vi "Kaelus PIM MeasParams TCP Cmds.vi"(1 "Option D?":bool, 4 "Legacy (f)?":bool, 6 "Force?":bool, 8 "error in":errorcluster, 9 "Measurement Parameters":T1={"IM Order"=0, "Averaging"=1, "Direction"=0, "Enable ALC?"=FALSE, "Enable SingleIM?"=FALSE, "Display Units"=enum."dBm", "VA Hold?"=FALSE, "DUT PORT"=enum."Port 1"} {"Direction" items=["Reverse", "Forward", "Auxiliary"]; "IM Order" items=["3rd", "5th", "7th", "9th", "11th", "13th", "15th", "17th", "19th", "21st", "23rd", "25th", "27th", "29th", "31st", "33rd"]; "Averaging" items=["None", "Minimum", "Normal", "High", "Maximum"]}) -> (0 "error out":errorcluster)   [LabVIEW 2011]
uses:
  PIM Cmd Params.ctl
  BPIMCore/HW IO/IMOrder.ctl
  BPIMCore/HW IO/HW Averaging.ctl
  BPIMCore/HW IO/MeasMode.ctl
  BPIMCore/Display/display_unit_format.ctl
  BPIMCore/HW IO/DUTport.ctl
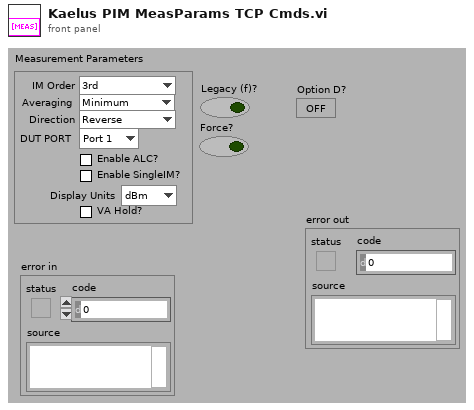
[diagram p1: front panel]
types:
  T1 = typedef "PIM Cmd Params.ctl" = cluster{"IM Order":T2, "Averaging":T3, "Direction":T4, "Enable ALC?":bool, "Enable SingleIM?":bool, "Display Units":T5, "VA Hold?":bool, "DUT PORT":T6}
  T2 = typedef "IMOrder.ctl" = u8
  T3 = typedef "HW Averaging.ctl" = u16
  T4 = typedef "MeasMode.ctl" = u16
  T5 = typedef "display_unit_format.ctl" = enum16{"dBm", "dBc"}
  T6 = typedef "DUTport.ctl" = enum16{"Port 1", "Port 2"}
  T7 = typedef "PIM.API.Command.Unique.ctl" = cluster{"#attributes":cluster{"Action":string}, "Double":dbl[], "Integer":i32[], "Boolean":bool[], "String":string[]}
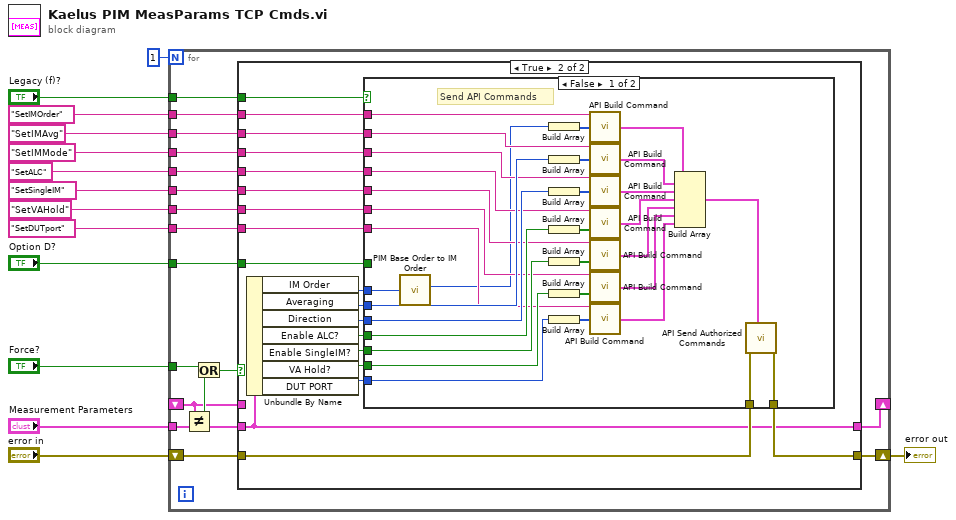
[diagram p0: block diagram]
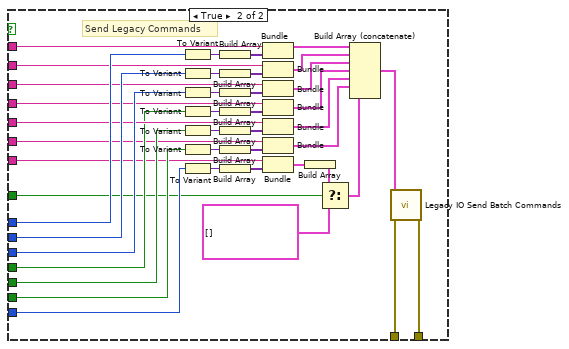
[diagram p3: hidden frame]
diagram:
  n1 = for {
    N: 1 -> [_]
    tunnel: "SetIMOrder" -> [w31]
    tunnel: "SetIMAvg" -> [w30]
    tunnel: "SetIMMode" -> [w29]
    tunnel: "SetALC" -> [w28]
    tunnel: "SetSingleIM" -> [w27]
    tunnel: "SetVAHold" -> [w26]
    tunnel: "SetDUTport" -> [w25]
    tunnel: "Option D?" -> [w24]
    shift-right: [w22] -> w5
    shift-left: "error in" -> [w23]
    shift-right: [w17] -> _
    shift-left: _ -> [w16]
    tunnel: "Measurement Parameters" -> [w19]
    tunnel: "Force?" -> [w20]
    tunnel: "Legacy (f)?" -> [w15]
    n2 = Not Equal?(x=w16, y=w19) -> (x != y?=w21:bool)
    n3 = Or(x=w20, y=w21) -> (x .or. y?=w18:bool)
    n4 = case shown="True" w18 {
      tunnel: w31 -> [_ w51]
      tunnel: w30 -> [_ w50]
      tunnel: w29 -> [_ w48]
      tunnel: w28 -> [_ w46]
      tunnel: w27 -> [_ w45]
      tunnel: w26 -> [_ w41]
      tunnel: w25 -> [_ w39]
      tunnel: w24 -> [_ w38]
      tunnel: w23 -> [w32 w37]
      tunnel: [w32 w36] -> w22
      tunnel: w19 -> [_ w35]
      tunnel: [w33 w35] -> w17
      tunnel: w16 -> [w33 _]
      tunnel: w15 -> [_ w34]
      frame False {
        # "No Changes have been made, proceed without sending commands."
      }
      frame True {
        n5 = Unbundle By Name(w35) -> ("IM Order"=w52:T2, "Averaging"=w49:T3, "Direction"=w47:T4, "Enable ALC?"=w44:bool, "Enable SingleIM?"=w43:bool, "VA Hold?"=w42:bool, "DUT PORT"=w40:T6)
        n6 = case shown="False" w34 {
          tunnel: w52 -> [w54 w126]
          tunnel: w51 -> [w84 w124]
          tunnel: w50 -> [w82 w121]
          tunnel: w49 -> [w81 w119]
          tunnel: w48 -> [w69 w117]
          tunnel: w47 -> [w79 w115]
          tunnel: w46 -> [w68 w113]
          tunnel: w45 -> [w67 w110]
          tunnel: w44 -> [w78 w108]
          tunnel: w43 -> [w77 w107]
          tunnel: w42 -> [w76 w106]
          tunnel: w41 -> [w66 w103]
          tunnel: w40 -> [w75 w102]
          tunnel: w39 -> [w65 w101]
          tunnel: w38 -> [_ w91]
          tunnel: w37 -> [w64 w86]
          tunnel: [w63 w85] -> w36
          frame False {
            # "Send API Commands"
            n7 = call "PIM Base Order to IM Order.vi"("Base Order (0)"=w54) -> ("IM Order"=w53:u8)  [unwired: 4 in, 1 out]
            n8 = Build Array(w53) -> (w83:u8[])
            n9 = Build Array(w81) -> (w80:T3[])
            n10 = Build Array(w79) -> (w70:T4[])
            n11 = Build Array(w78) -> (w71:bool[])
            n12 = Build Array(w77) -> (w72:bool[])
            n13 = Build Array(w76) -> (w73:bool[])
            n14 = Build Array(w75) -> (w74:T6[])
            n15 = call "API Build Command.vi"("Action"=w84, "Integer"=w83) -> ("PIM.API.Command.Unique"=w62:T7)  [unwired: 13 in]
            n16 = call "API Build Command.vi"("Action"=w82, "Integer"=w80) -> ("PIM.API.Command.Unique"=w61:T7)  [unwired: 13 in]
            n17 = call "API Build Command.vi"("Action"=w69, "Integer"=w70) -> ("PIM.API.Command.Unique"=w60:T7)  [unwired: 13 in]
            n18 = call "API Build Command.vi"("Action"=w68, "Boolean"=w71) -> ("PIM.API.Command.Unique"=w59:T7)  [unwired: 13 in]
            n19 = call "API Build Command.vi"("Action"=w67, "Boolean"=w72) -> ("PIM.API.Command.Unique"=w58:T7)  [unwired: 13 in]
            n20 = call "API Build Command.vi"("Action"=w66, "Boolean"=w73) -> ("PIM.API.Command.Unique"=w57:T7)  [unwired: 13 in]
            n21 = call "API Build Command.vi"("Action"=w65, "Integer"=w74) -> ("PIM.API.Command.Unique"=w56:T7)  [unwired: 13 in]
            n22 = Build Array(w62, w61, w60, w59, w58, w57, w56) -> (w55:T7[])
            n23 = call "API Send Authorized Commands.vi"("Commands"=w55, "error in (no error)"=w64) -> ("error out"=w63:errorcluster)  [unwired: 7 in, 2 out]
          }
          frame True {
            # "Send Legacy Commands"
            n24 = To Variant(anything=w126) -> (Variant=w125:variant)
            n25 = To Variant(anything=w119) -> (Variant=w120:variant)
            n26 = To Variant(anything=w115) -> (Variant=w118:variant)
            n27 = To Variant(anything=w108) -> (Variant=w112:variant)
            n28 = To Variant(anything=w107) -> (Variant=w111:variant)
            n29 = To Variant(anything=w106) -> (Variant=w105:variant)
            n30 = To Variant(anything=w102) -> (Variant=w99:variant)
            n31 = Build Array(w125) -> (w123:variant[])
            n32 = Build Array(w120) -> (w122:variant[])
            n33 = Build Array(w118) -> (w116:variant[])
            n34 = Build Array(w112) -> (w114:variant[])
            n35 = Build Array(w111) -> (w109:variant[])
            n36 = Build Array(w105) -> (w104:variant[])
            n37 = Build Array(w99) -> (w100:variant[])
            n38 = Bundle(w124, w123) -> (w97:cluster{string, variant[]})  [unwired: 1 out]
            n39 = Bundle(w121, w122) -> (w96:cluster{string, variant[]})  [unwired: 1 out]
            n40 = Bundle(w117, w116) -> (w95:cluster{string, variant[]})  [unwired: 1 out]
            n41 = Bundle(w113, w114) -> (w94:cluster{string, variant[]})  [unwired: 1 out]
            n42 = Bundle(w110, w109) -> (w93:cluster{string, variant[]})  [unwired: 1 out]
            n43 = Bundle(w103, w104) -> (w92:cluster{string, variant[]})  [unwired: 1 out]
            n44 = Bundle(w101, w100) -> (w98:cluster{string, variant[]})  [unwired: 1 out]
            n45 = Build Array(w98) -> (w90:cluster{string, variant[]}[])
            n46 = Select(t=w90, s=w91, f=cluster{string, variant[]}[] []) -> (s? t:f=w88:cluster{string, variant[]}[])
            n47 = Build Array (concatenate)(w97, w96, w95, w94, w93, w92, w88) -> (w87:cluster{string, variant[]}[])
            n48 = call "Legacy IO Send Batch Commands.vi"("error in"=w86, "Legacy Commands Array"=w87) -> ("error out"=w85:errorcluster)  [unwired: 9 in]
          }
        }
      }
    }
  }
  "error out" <- w5
